vi "MU Set Register.vi"(7 "writeVerify":u32, 8 "error in (no error)":errorcluster, 9 "value":u32, 10 "address":u32, 11 "handle":u64) -> (0 "error out (no error)":errorcluster, 3 "function return":u32)   [LabVIEW 2017, in "MU_3SL_interface.lvlib"]
uses:
  MU_3SL_interface.lvlib
  lib/MU_3SL_interface.dll
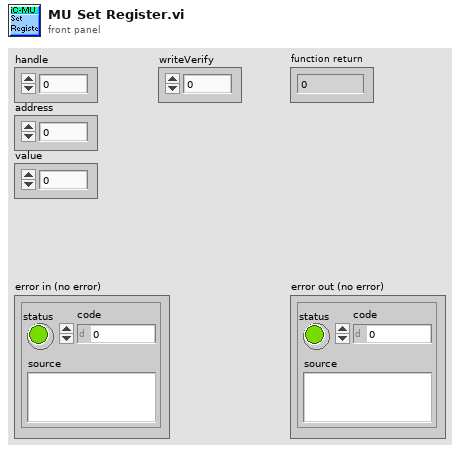
[diagram p1: front panel]
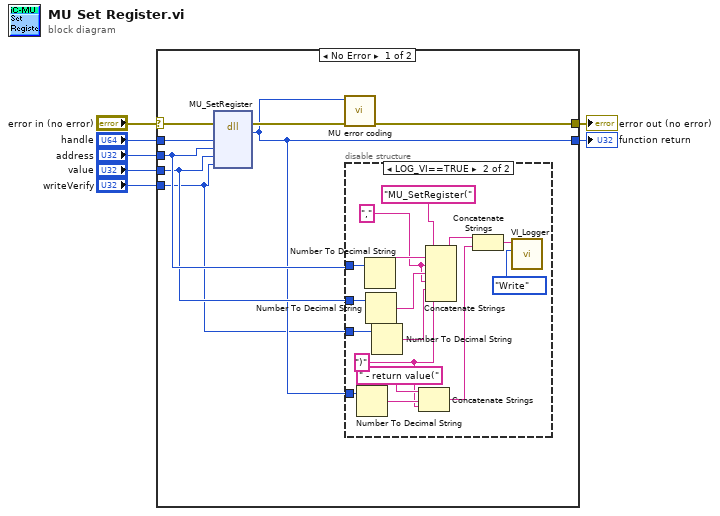
[diagram p0: block diagram]
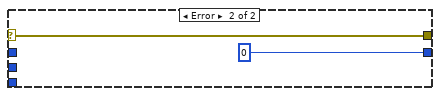
[diagram p3: hidden frame]
diagram:
  n1 = case shown="No Error" "error in (no error)" {
    selector: "error in (no error)" -> [w12 w33]
    tunnel: [w9 u32 0] -> w7
    tunnel: "handle" -> [w15 _]
    tunnel: "address" -> [w11 _]
    tunnel: "value" -> [w10 _]
    tunnel: "writeVerify" -> [w8 _]
    tunnel: [w13 w33] -> w2
    frame No Error {
      n2 = dll-call lib="C:/Users/bes/AppData/Roaming/work/mu_9so/icsubmodules/soft_mu_3sl_master/lv_interface/lib/MU_3SL_interface**.*" fn="MU_SetRegister"(error in=w12, "handle"=w15, "address"=w11, "value"=w10, "writeVerify"=w8) -> (error out=w14:errorcluster, "return type"=w9:u32)  [unwired: 6 in, 1 out]
      n3 = call "MU error coding.vi"("error in (no error)"=w14, "function return in"=w9) -> ("error out"=w13:errorcluster)  [unwired: 9 in]
      n4 = disable-structure shown="LOG_VI==TRUE" {
        disable-tunnel: w9 -> [_ w29]
        disable-tunnel: w11 -> [_ w24]
        disable-tunnel: w10 -> [_ w22]
        disable-tunnel: w8 -> [_ w18]
        frame condition #0 {
        }
        frame condition #1 (active) {
          w16 = ")" ("string")
          w19 = "," ("string")
          n5 = Number To Decimal String(number=w29) -> (decimal integer string=w28:string)  [unwired: 1 in]
          n6 = Number To Decimal String(number=w24) -> (decimal integer string=w23:string)  [unwired: 1 in]
          n7 = Number To Decimal String(number=w22) -> (decimal integer string=w21:string)  [unwired: 1 in]
          n8 = Number To Decimal String(number=w18) -> (decimal integer string=w17:string)  [unwired: 1 in]
          n9 = Concatenate Strings(" - return value(" ("string"), w28, w16) -> (w26:string)
          n10 = Concatenate Strings("MU_SetRegister(" ("Info in"), w23, w19, w21, w19, w17, w16) -> (w27:string)
          n11 = Concatenate Strings(w27, w26) -> (w25:string)
          n12 = call "VI_Logger.vi"("Action (Read)"=enum16{"Write", "Read"}."Write", "Info in"=w25) -> ()  [unwired: 8 in, 2 out]
        }
      }
    }
    frame Error {
    }
  }
  "function return" <- w7
  "error out (no error)" <- w2
